vi "SDI-12 Continuous Operations.vi"(0 "RS232 Port In":refnum<visa-resource-name>="COM11", 1 "Sensor Address In":string="0", 2 "Cumulative Volume":dbl, 3 "Sonde Data Ctl Refnum":refnum<vi>, 4 "Stop Ctl Refnum":refnum<vi>, 5 "Error In (No Error)":errorcluster, 6 "file directory (dialog if empty)":path=path "D:/Cascade/Raw Data files", 7 "Save File":bool) -> (11 "Measurements Out":dbl[](array[numeric]), 12 "new file path (Not A Path if cancelled)":path, 13 "Array":timestamp[](array[timestamp]), 15 "Address Out":string="a" caption="sensor address out", 16 "output cluster":T1 caption="Cluster" {"Salinity" format="%_3g"; "Temp" format="%_2g"; "ORP" format="%_4g"; "pH" format="%_4g"; "Dissolved\nOxygen" format="%_4g"; "Specific\nConductance" format="%_4g"; "Cumulative\nVolume" format="%#_4g"}, 17 "Temperature":cluster{"Y":dbl[], "Y":dbl[]}[](graph), 18 "Sonde Data Display":T2, 19 "Error Out":errorcluster)   [LabVIEW 2016]
doc: "A general set of examples of the SDI-12 API for a generic sensor. A tab control separates each example, and contains the following examples:\n1. Read Single.\n2. Read Multiple.\n3. Acknowledge Active.\n4. Change Address.\n5. Address Query.\n6. Send Identification."
uses:
  SDI-12/Sonde Vertical Graph.ctl
  Waterloo DAQ/controls/Vertical Chart.ctl
  activeXtest/activeXtest 2015 Folder/sonde cluster.ctl
  <vilib>/Utility/file.llb/Write Delimited Spreadsheet (string).vi
  <vilib>/Utility/file.llb/Write Delimited Spreadsheet (DBL).vi
  SDI-12/SDI-12.lvlib
panel:
  out "Sensor On/Off Response":bool
  out "Battery Voltage (V)":dbl
  out "Number of Measurements Out":i32
  in  "Measurement Type In (Normal)":i32(ring)=1 items=["Normal", "Concurrent", "Continuous"]
  out "Parameter Out":i32(ring) items=["0", "1", "2", "3", "4", "5", "6", "7", "8", "9"]
  in  "Parameter In (0)":i32(ring) items=["0", "1", "2", "3", "4", "5", "6", "7", "8", "9"]
  in  "CRC (False)":bool
  out "CRC Out":bool
  out "Measurement Type Out":i32(ring) items=["Normal", "Concurrent", "Continuous"]
  out "Time (s)":dbl
  in  "stop":bool
  out "counter":i32
  out "start time":timestamp
  # "deg C"
  # "pH"
  # "specific conductance"
  # "salinity"
  # "DO % saturation"
  # "DO mg/L"
  # "ORP"
  # "depth"
  # "battery"
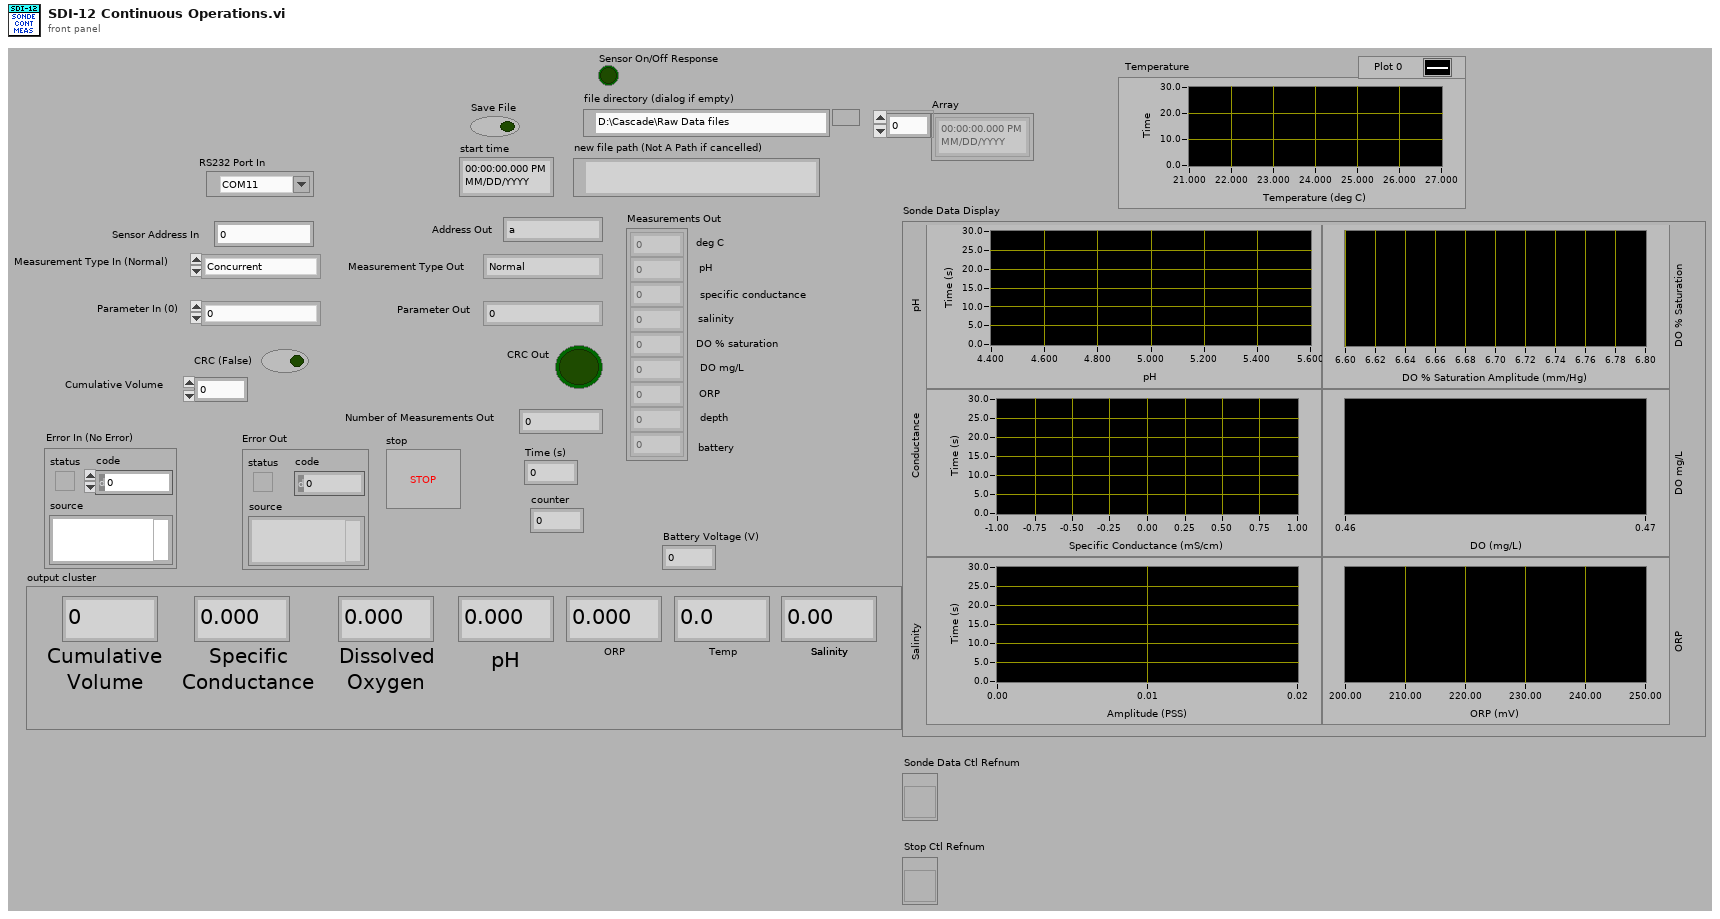
[diagram p1: front panel]
types:
  T1 = typedef "sonde cluster.ctl" = cluster{"Cumulative\nVolume":dbl, "Specific\nConductance":dbl, "Dissolved\nOxygen":dbl, "pH":dbl, "ORP":dbl, "Temp":dbl, "Salinity":dbl}
  T2 = typedef "Sonde Vertical Graph.ctl" = cluster{"pH":T3, "Conductance":T3, "Salinity":T3, "DO % Saturation":T3, "DO mg/L":T3, "ORP":T3}
  T3 = typedef "Vertical Chart.ctl" = cluster{"Y":dbl[], "Y":dbl[]}[]
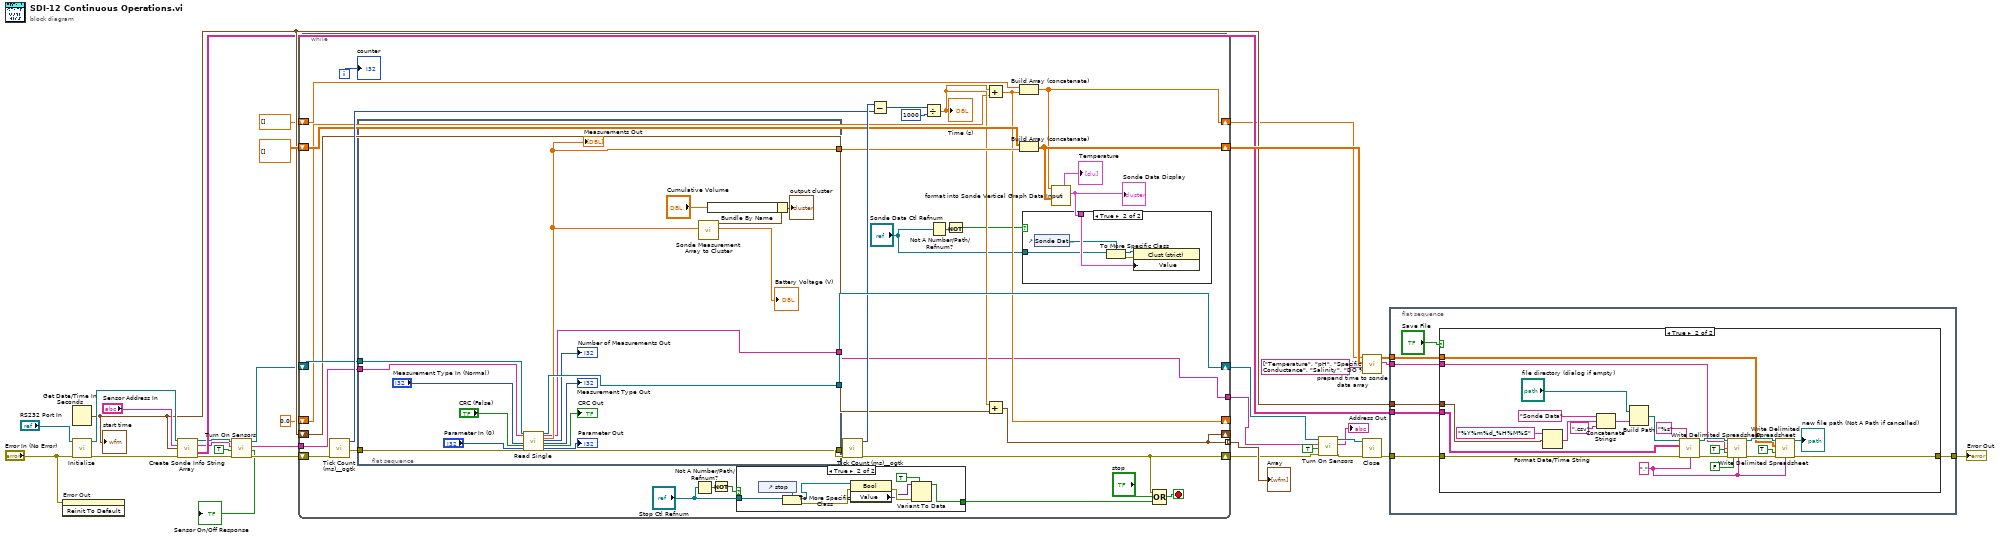
[diagram p0: block diagram]
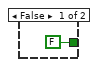
[diagram p3: hidden frame]
diagram:
  n1 = invoke on="Error Out" class="Clust (strict)" method="Reinit To Default"(error in="Error In (No Error)") -> ()  [unwired: 2 in, 3 out]
  n2 = Get Date/Time In Seconds() -> (seconds since 1Jan1904=w23:timestamp)
  "start time" <- w23
  n3 = call "Initialize.vi"("Error In (No Error)"="Error In (No Error)", "RS232 Port In"="RS232 Port In") -> ("Error Out"=w32:errorcluster, "RS232 Port Out"=w31:refnum<visa-resource-name>)  [unwired: 8 in]
  n4 = call "Create Sonde Info String Array.vi"("VISA Refnum in"=w31, "Sensor Address In"="Sensor Address In", "seconds since 1Jan1904"=w23, "error in (no error)"=w32) -> ("VISA Refnum out"=w14:refnum<visa-resource-name>, "Address Out"=w12:string, "Array"=w22:string[][], "error out"=w16:errorcluster)  [unwired: 8 in]
  n5 = call "Turn On Sensors.vi"("Error In (No Error)"=w16, "Sensor On/Off"=TRUE, "Sensor Address In"=w12, "RS232 Port In"=w14) -> ("Error Out"=w15:errorcluster, "Sensor On/Off Response"=→"Sensor On/Off Response":bool, "Address Out"=w11:string, "RS232 Port Out"=w13:refnum<visa-resource-name>)  [unwired: 4 in]
  n6 = while {
    shift-right: [w67] -> w7
    shift-left: w13 -> [w60]
    shift-right: [w43] -> w9
    shift-left: w15 -> [w59]
    shift-right: [w54] -> w28
    shift-left: dbl[][] [] -> [w55]
    tunnel: [w52] -> w29 mode=indexing
    shift-right: [w52] -> _
    shift-left: w23 -> [w53]
    shift-right: [w50] -> w19
    shift-left: dbl[] [] -> [w47]
    tunnel: w11 -> [w51]
    shift-right: [w46] -> _
    shift-left: 0.0 -> [w48]
    tunnel: [w42] -> w5
    i -> [w57]
    stop <- w44 stop-if-true
    n7 = call <userlib>:"Tick Count (ms)__ogtk.vi"("error in (no error)"=w59) -> ("error out"=w65:errorcluster, "millisecond timer value"=w63:u32)  [unwired: 9 in]
    n8 = flat-sequence {
      tunnel: [w99] -> w67
      tunnel: [w98] -> w66
      tunnel: w65 -> [w90]
      tunnel: w60 -> [w89]
      tunnel: [w87] -> w56
      tunnel: w51 -> [w88]
      tunnel: [w86] -> w42
      frame #0 {
        n9 = call "Read Single.vi"("RS232 Port In"=w89, "Sensor Address In"=w88, "Measurement Type In (Normal)"="Measurement Type In (Normal)", "CRC (False)"="CRC (False)", "Parameter In (0)"="Parameter In (0)", "Error In (No Error)"=w90) -> ("RS232 Port Out"=w99:refnum<visa-resource-name>, "Sensor Address Out"=w86:string, "Measurements Out"=w87:dbl[], "Number of Measurements Out"=→"Number of Measurements Out":i32, "Measurement Type Out"=→"Measurement Type Out":i32, "CRC Out"=→"CRC Out":bool, "Parameter Out"=→"Parameter Out":i32, "Error Out"=w98:errorcluster)  [unwired: 14 in]
        "Measurements Out" <- w87
        n10 = call "Sonde Measurement Array to Cluster.vi"("Measurements In"=w87) -> ("Battery Voltage (V)"=→"Battery Voltage (V)":dbl, "Sonde Data Cluster"=w83:T1)  [unwired: 9 in]
        n11 = Bundle By Name(cluster=w83, "Cumulative\nVolume"="Cumulative Volume") -> (→"output cluster":T1)
      }
    }
    n12 = Not A Number/Path/Refnum?(number/path/refnum="Stop Ctl Refnum") -> (NaN/Path/Refnum?=w37:bool)
    n13 = Not(x=w37) -> (.not. x?=w35:bool)
    n14 = case shown="True" w35 {
      tunnel: "Stop Ctl Refnum" -> [_ w76]
      tunnel: [FALSE w69] -> w34
      frame False {
      }
      frame True {
        n15 = control-ref of="stop"() -> (w74:refnum<vi>)
        n16 = To More Specific Class(target class=w74, reference=w76) -> (specific class reference=w71:refnum<vi>, error out=w75:errorcluster)  [unwired: 1 in]
        n17 = property class="Bool"(reference=w71, error in=w75) -> (error out=w73:errorcluster, "Value"=w72:variant)  [unwired: 1 out]
        n18 = Variant To Data(error in=w73, type=TRUE, Variant=w72) -> (data=w69:bool)  [unwired: 1 out]
      }
    }
    n19 = call <userlib>:"Tick Count (ms)__ogtk.vi"("error in (no error)"=w66) -> ("error out"=w43:errorcluster, "millisecond timer value"=w64:u32)  [unwired: 9 in]
    n20 = Subtract(x=w64, y=w63) -> (x-y=w62:u32)
    n21 = Divide(x=w62, y=u32 1000) -> (x/y=w49:dbl)
    "Time (s)" <- w49
    n22 = Not A Number/Path/Refnum?(number/path/refnum="Sonde Data Ctl Refnum") -> (NaN/Path/Refnum?=w41:bool)
    n23 = Not(x=w41) -> (.not. x?=w40:bool)
    n24 = Add(x=w49, y=w48) -> (x+y=w46:dbl)
    n25 = Add(x=w49, y=w53) -> (x+y=w52:timestamp)
    n26 = Build Array (concatenate)(w47, w46) -> (w50:dbl[])
    n27 = Build Array (concatenate)(w55, w56) -> (w54:dbl[][])
    n28 = call "format into Sonde Vertical Graph Data Input.vi"("Sonde Measurement Array"=w54, "Time Array"=w50) -> ("Sonde Data Display"=w39:T2, "Temperature"=→"Temperature":cluster{"X":dbl[], "Y":dbl[]}[])  [unwired: 8 in]
    "Sonde Data Display" <- w39
    n29 = case shown="True" w40 {
      tunnel: w39 -> [_ w81]
      tunnel: "Sonde Data Ctl Refnum" -> [_ w79]
      frame False {
      }
      frame True {
        n30 = control-ref of="Sonde Data Display"() -> (w80:refnum<vi>)
        n31 = To More Specific Class(target class=w80, reference=w79) -> (specific class reference=w78:refnum<vi>, error out=w77:errorcluster)  [unwired: 1 in]
        n32 = property class="Clust (strict)"(reference=w78, error in=w77, "Value"=w81) -> ()  [unwired: 2 out]
      }
    }
    n33 = Compound Arithmetic op=OR(w43, "stop", w34) -> (w44:bool)
    "counter" <- w57
  }
  "Array" <- w29
  n34 = call "Turn On Sensors.vi"("Error In (No Error)"=w9, "Sensor On/Off"=TRUE, "Sensor Address In"=w5, "RS232 Port In"=w7) -> ("Error Out"=w8:errorcluster, "Address Out"=→"Address Out":string, "RS232 Port Out"=w6:refnum<visa-resource-name>)  [unwired: 4 in, 1 out]
  n35 = call "prepend time to sonde data array.vi"("Measurement Labels"=string[] ["Temperature", "pH", "Specific Conductance", "Salinity", "DO % saturation", "DO", "ORP", "depth", "battery"], "Sonde\nData Array"=w28, "Time Array"=w19) -> ("Header Array"=w21:string[], "Data Array"=w25:dbl[][])  [unwired: 7 in]
  n36 = call "Close.vi"("Error In (No Error)"=w8, "RS232 Port In"=w6) -> ("Error Out"=w27:errorcluster)  [unwired: 9 in]
  n37 = flat-sequence {
    tunnel: w27 -> [w106]
    tunnel: [w105] -> w26
    tunnel: w21 -> [w103]
    tunnel: w25 -> [w102]
    tunnel: w23 -> [w101]
    tunnel: w22 -> [w100]
    frame #0 {
      n38 = case shown="True" "Save File" {
        tunnel: [w107 w127] -> w105
        tunnel: w106 -> [w107 w112]
        tunnel: w103 -> [_ w108]
        tunnel: w102 -> [_ w125]
        tunnel: w101 -> [_ w119]
        tunnel: w100 -> [_ w110]
        frame False {
        }
        frame True {
          w109 = "," ("delimiter (\\t)")
          n39 = Format Date/Time String(time format string (%c)="%Y%m%d_%H%M%S", seconds (now)=w119) -> (date/time string=w118:string)  [unwired: 1 in]
          n40 = Concatenate Strings("Sonde Data" ("name or relative path"), w118, ".csv" ("string")) -> (w120:string)
          n41 = Build Path(base path="file directory (dialog if empty)", name or relative path=w120) -> (appended path=w115:path)
          n42 = call-poly <vilib>:"Write Delimited Spreadsheet.vi"("file path (dialog if empty)"=w115, "format (%s)"="%s" ("format (%.3f)"), "2D data"=w110, "error in (no error)"=w112, "delimiter (\\t)"=w109) -> ("new file path (Not A Path if cancelled)"=w114:path, "error out"=w111:errorcluster)  [unwired: 9 in]
          n43 = call-poly <vilib>:"Write Delimited Spreadsheet.vi"("file path (dialog if empty)"=w114, "1D data"=w108, "append to file? (new file:F)"=TRUE ("append to file? (F)"), "error in (no error)"=w111, "transpose? (no:F)"=FALSE ("transpose? (F)"), "delimiter (\\t)"=w109) -> ("new file path (Not A Path if cancelled)"=w129:path, "error out"=w128:errorcluster)  [unwired: 8 in]
          n44 = call-poly <vilib>:"Write Delimited Spreadsheet.vi"("file path (dialog if empty)"=w129, "2D data"=w125, "append to file? (new file:F)"=TRUE ("append to file? (F)"), "error in (no error)"=w128, "delimiter (\\t)"=w109) -> ("new file path (Not A Path if cancelled)"=→"new file path (Not A Path if cancelled)":path, "error out"=w127:errorcluster)  [unwired: 9 in]
        }
      }
    }
  }
  "Error Out" <- w26
